vi "Radio Number Generator.vi"(11 "Adjacency Matrix":T1) -> (1 "Start Value":i32, 2 "Radio Number":i32, 3 "Run Time ms":u32)   [LabVIEW 2016]
uses:
  <vilib>/Analysis/Matrix/Datatypes/RealMatrix.ctl
  <vilib>/Analysis/Matrix/NI_Matrix.lvlib
panel:
  out "Labelings":i32[][](array[numeric])
  out "N":i32
  out "Radio Numbers":i32[](array[numeric])
  in  "Thereotical Maximum (if zero computed for all graphs)":dbl
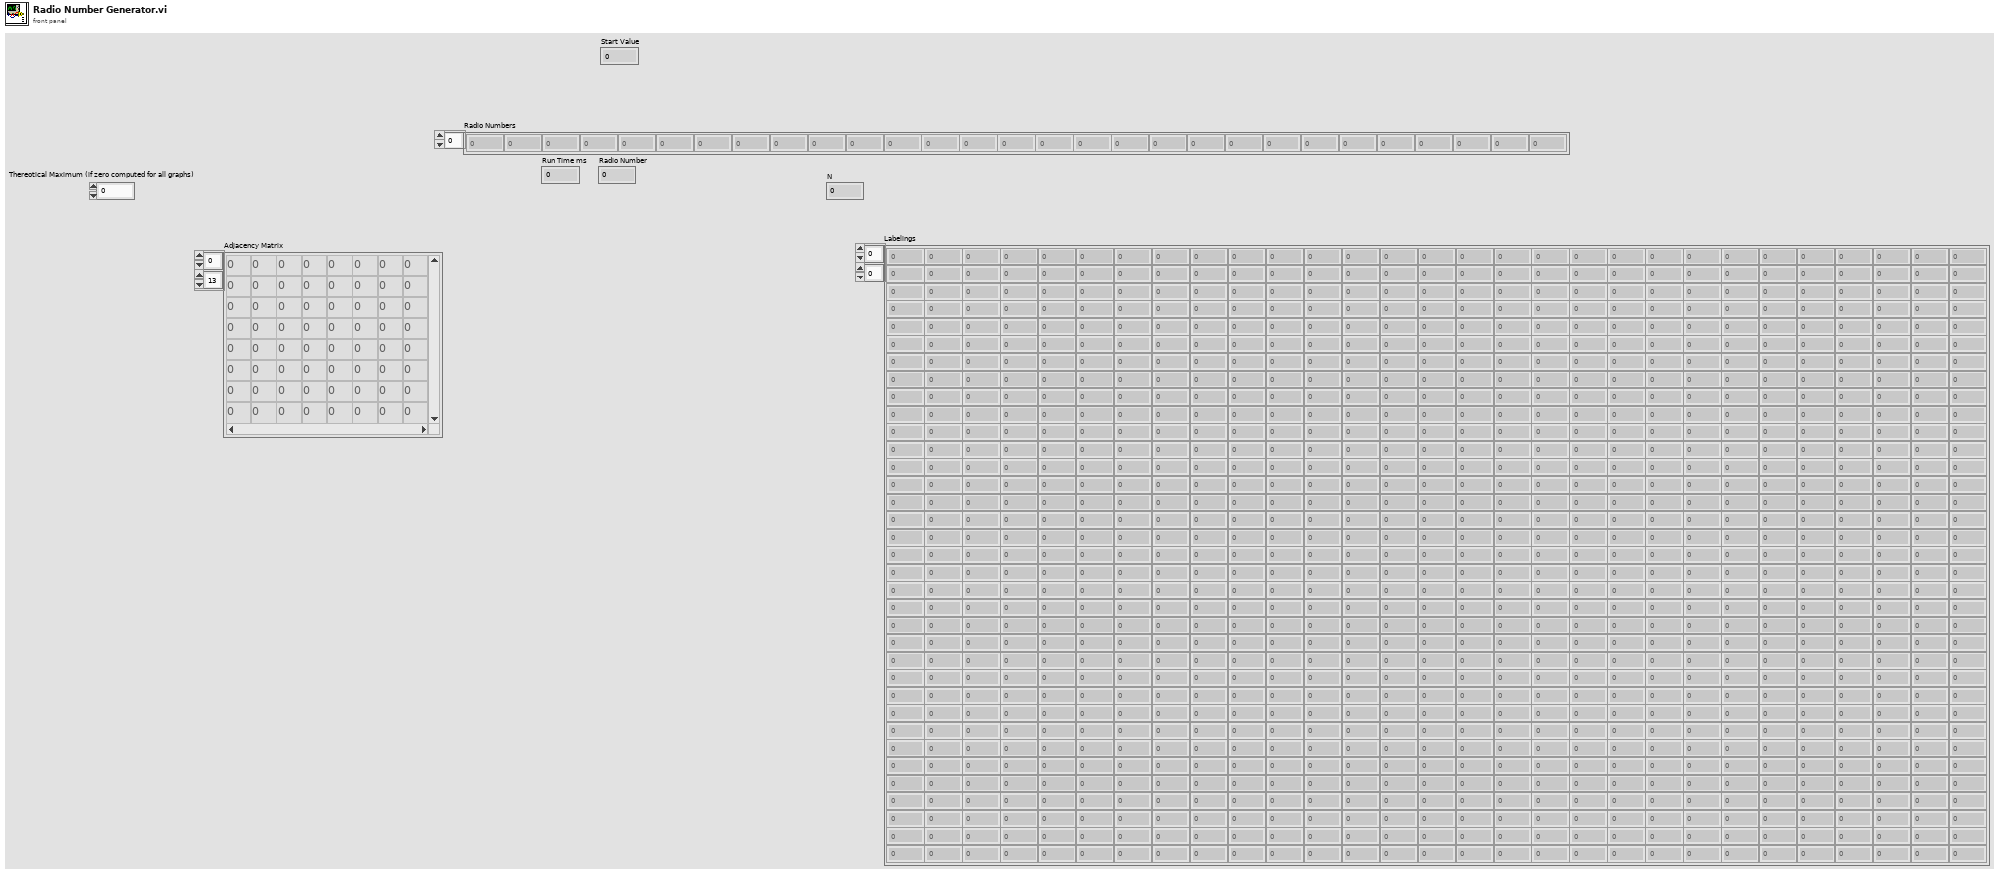
[diagram p1: front panel]
types:
  T1 = typedef "NI_Matrix.lvlib/RealMatrix.ctl" = dbl[][]
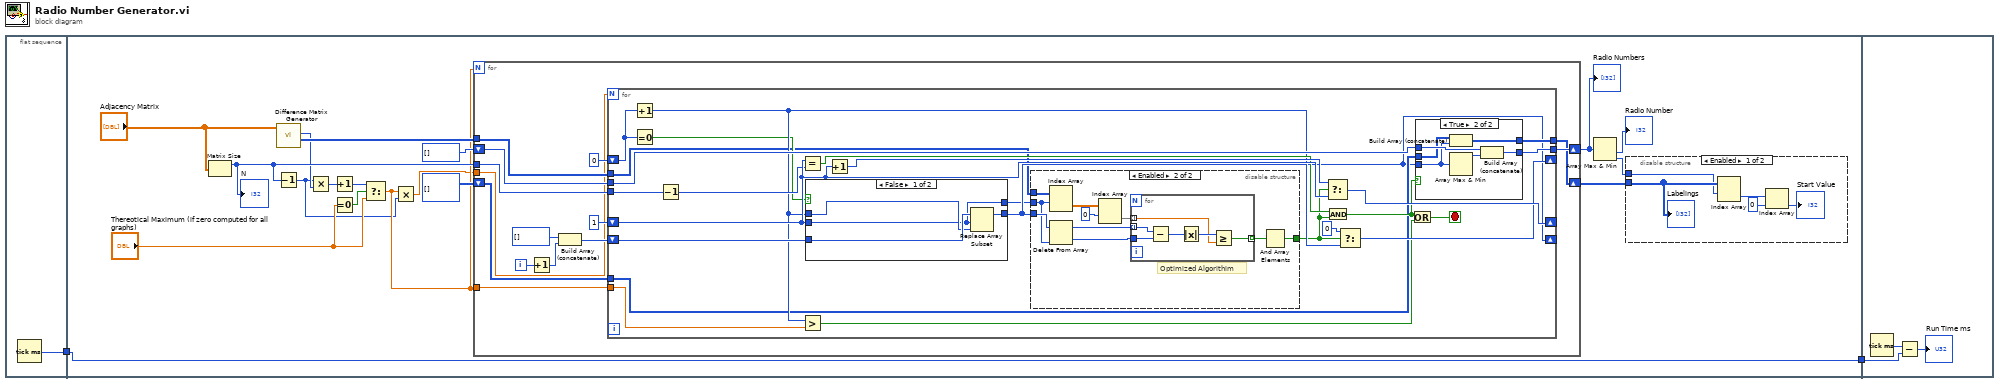
[diagram p0: block diagram]
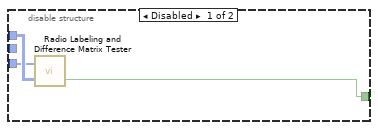
[diagram p3: hidden frame]
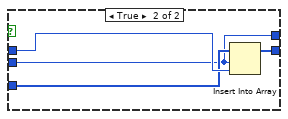
[diagram p4: hidden frame]
diagram:
  n1 = flat-sequence {
    tunnel: [w3] -> w1
    tunnel: [w19] -> w2
    tunnel: w1 -> [w19]
    tunnel: w2 -> [w101]
    frame #0 {
      n2 = Tick Count (ms)() -> (millisecond timer value=w3:u32)
    }
    frame #1 {
      n3 = Matrix Size(0:"Adjacency Matrix") -> (1:w15:i32)  [unwired: 1 out]
      "N" <- w15
      n4 = call "Difference Matrix Generator.vi"("Adjacency Matrix"="Adjacency Matrix") -> ("Difference Matrix"=w21:i32[][], "Diameter"=w14:i32)  [unwired: 8 in, 1 out]
      n5 = Decrement(x=w15) -> (x-1=w7:i32)
      n6 = Multiply(x=w7, y=w14) -> (x*y=w13:i32)
      n7 = Increment(x=w13) -> (x+1=w16:i32)
      n8 = Equal To 0?(x="Thereotical Maximum (if zero computed for all graphs)") -> (x = 0?=w18:bool)
      n9 = Select(t=w16, s=w18, f="Thereotical Maximum (if zero computed for all graphs)") -> (s? t:f=w8:dbl)
      n10 = Multiply(x=w8, y=w7) -> (x*y=w6:dbl)
      n11 = for {
        N: w8 -> [_]
        tunnel: w21 -> [w30]
        tunnel: w15 -> [w38]
        tunnel: w8 -> [w33]
        shift-right: [w31] -> w12
        shift-left: i32[] [] -> [w32]
        shift-right: [w29] -> w10
        shift-left: i32[][] [] -> [w28]
        tunnel: w6 -> [w27]
        i -> [w35]
        n12 = Increment(x=w35) -> (x+1=w34:i32)
        n13 = Build Array (concatenate)(i32[] [], w34) -> (w36:i32[])
        n14 = for {
          N: w27 -> [_]
          tunnel: w30 -> [w42]
          shift-right: [w63] -> _
          shift-left: 1 -> [w60]
          shift-right: [w44] -> _
          shift-left: w36 -> [w52]
          shift-right: [w62] -> _
          shift-left: 0 -> [w49]
          tunnel: w38 -> [w59]
          tunnel: w33 -> [w56]
          tunnel: w32 -> [w53]
          tunnel: [w51] -> w31
          tunnel: [w47] -> w29
          tunnel: w28 -> [w46]
          stop <- w45 stop-if-true
          n15 = Increment(x=w49) -> (x+1=w50:i32)
          n16 = Equal To 0?(x=w49) -> (x = 0?=w48:bool)
          n17 = Decrement(x=w59) -> (x-1=w58:i32)
          n18 = Equal?(x=w60, y=w58) -> (x = y?=w57:bool)
          n19 = Greater?(x=w50, y=w56) -> (0:w55:bool)
          n20 = case shown="False" w48 {
            tunnel: w60 -> [w84 w88]
            tunnel: w52 -> [w87 w89]
            tunnel: [w86 w91] -> w44
            tunnel: w50 -> [w85 w90]
            tunnel: [w84 w88] -> w43
            frame False {
              n21 = Replace Array Subset(array=w87, new element=w85, index=w84) -> (w86:i32[])
            }
            frame True {
              n22 = Insert Into Array(array=w89, index=w88, new element=w90) -> (w91:i32[])
            }
          }
          n23 = Increment(x=w60) -> (x+1=w64:i32)
          n24 = disable-structure shown="Enabled" {
            disable-tunnel: w42 -> [w67 w77]
            disable-tunnel: [w66 w68] -> w41
            disable-tunnel: w44 -> [w65 w76]
            disable-tunnel: w43 -> [_ w75]
            frame Disabled {
              n25 = call "Radio Labeling and Difference Matrix Tester.vi"("Difference Between Labels Matrix"=w67, "Radio Labels"=w65) -> ("Works?"=w66:bool)  [unwired: 1 out]
            }
            frame Enabled {
              # "Optimized Algorithim"
              n26 = Index Array(array=w77, index (row)=w75) -> (element=w71:dbl[][])  [unwired: 1 in]
              n27 = Delete From Array(array=w76, index=w75) -> (deleted portion=w74:i32, array with subset deleted=w73:i32[])  [unwired: 1 in]
              n28 = Index Array(array=w71, index (row)=0) -> (element=w69:dbl[])  [unwired: 1 in]
              n29 = for {
                tunnel: w74 -> [w80]
                tunnel: w73 -> [w81] mode=indexing
                tunnel: w69 -> [w79] mode=indexing
                tunnel: [w78] -> w72 mode=indexing
                n30 = Subtract(x=w81, y=w80) -> (x-y=w83:i32)
                n31 = Absolute Value(x=w83) -> (abs(x)=w82:i32)
                n32 = Greater Or Equal?(x=w82, y=w79) -> (x >= y?=w78:bool)
              }
              n33 = And Array Elements(Boolean array=w72) -> (logical AND=w68:bool)
            }
          }
          n34 = Select(t=w64, s=w41, f=w60) -> (s? t:f=w63:i32)
          n35 = And(x=w57, y=w41) -> (x .and. y?=w54:bool)
          n36 = Select(t=0, s=w41, f=w50) -> (s? t:f=w62:i32)
          n37 = Or(x=w54, y=w55) -> (x .or. y?=w45:bool)
          n38 = case shown="True" w54 {
            tunnel: w53 -> [w93 w99]
            tunnel: w44 -> [_ w94]
            tunnel: [w93 w97] -> w51
            tunnel: [w92 w96] -> w47
            tunnel: w46 -> [w92 w95]
            frame False {
            }
            frame True {
              n39 = Build Array (concatenate)(w95, w94) -> (w96:i32[][])
              n40 = Array Max & Min(array=w94) -> (max value=w98:i32)  [unwired: 3 out]
              n41 = Build Array (concatenate)(w99, w98) -> (w97:i32[])
            }
          }
        }
      }
      "Radio Numbers" <- w12
      n42 = Array Max & Min(array=w12) -> (min value=→"Radio Number":i32, min index (indices)=w4:i32)  [unwired: 2 out]
      n43 = disable-structure shown="Enabled" {
        disable-tunnel: w10 -> [w26 _]
        disable-tunnel: w4 -> [w25 _]
        frame Enabled {
          n44 = Index Array(array=w26, index (row)=w25) -> (element=w24:i32[])  [unwired: 1 in]
          n45 = Index Array(array=w24, index=0) -> (element=→"Start Value":i32)
          "Labelings" <- w26
        }
        frame Disabled {
        }
      }
    }
    frame #2 {
      n46 = Tick Count (ms)() -> (millisecond timer value=w102:u32)
      n47 = Subtract(x=w102, y=w101) -> (x-y=→"Run Time ms":u32)
    }
  }
